vi "initCSMs.vi"(7 "Enable building lvlibp?":bool, 8 "error in (no error)":errorcluster, 11 "TestCase in":refnum<class "testcase-CSMAddonLoopSupport.lvclass">) -> (0 "error out":errorcluster, 3 "TestCase out":refnum<class "testcase-CSMAddonLoopSupport.lvclass">)   [LabVIEW 2017, in "testcase-CSMAddonLoopSupport.lvclass"]
uses:
  testcase-CSMAddonLoopSupport.lvclass
  testcase-CSMAddonLoopSupport.lvclass/testcase-CSMAddonLoopSupport.ctl
  CSM/Normal-CSM.vi
  <vilib>/AppBuilder/AB_API_Simple/Build (path).vi
  CSM/Chain1.vi
  CSM/Chain2.vi
  CSM/Chain3.vi
  <vilib>/addons/_JKI Toolkits/VI Tester/TestCase.llb/TestCase.lvclass
  CSM/CSM-Testcase.lvlib
  src/user.lib/_NEVSTOP/Communicable State Machine(CSM)/Communicable State Machine.lvlib
  <vilib>/AppBuilder/AB_API_Simple/NI_App_Builder_API.lvlib
  C:/Program Files (x86)/National Instruments/LabVIEW 2017/vi.lib/addons/_JKI Toolkits/VI Tester/TestCase.llb/TestCase.lvclass
panel:
  out "CSMs":string[](array[string])
  out "Generated files":path[](array[path])
  out "CSMs Left":string[](array[string])
  out "Waited (ms)":u32
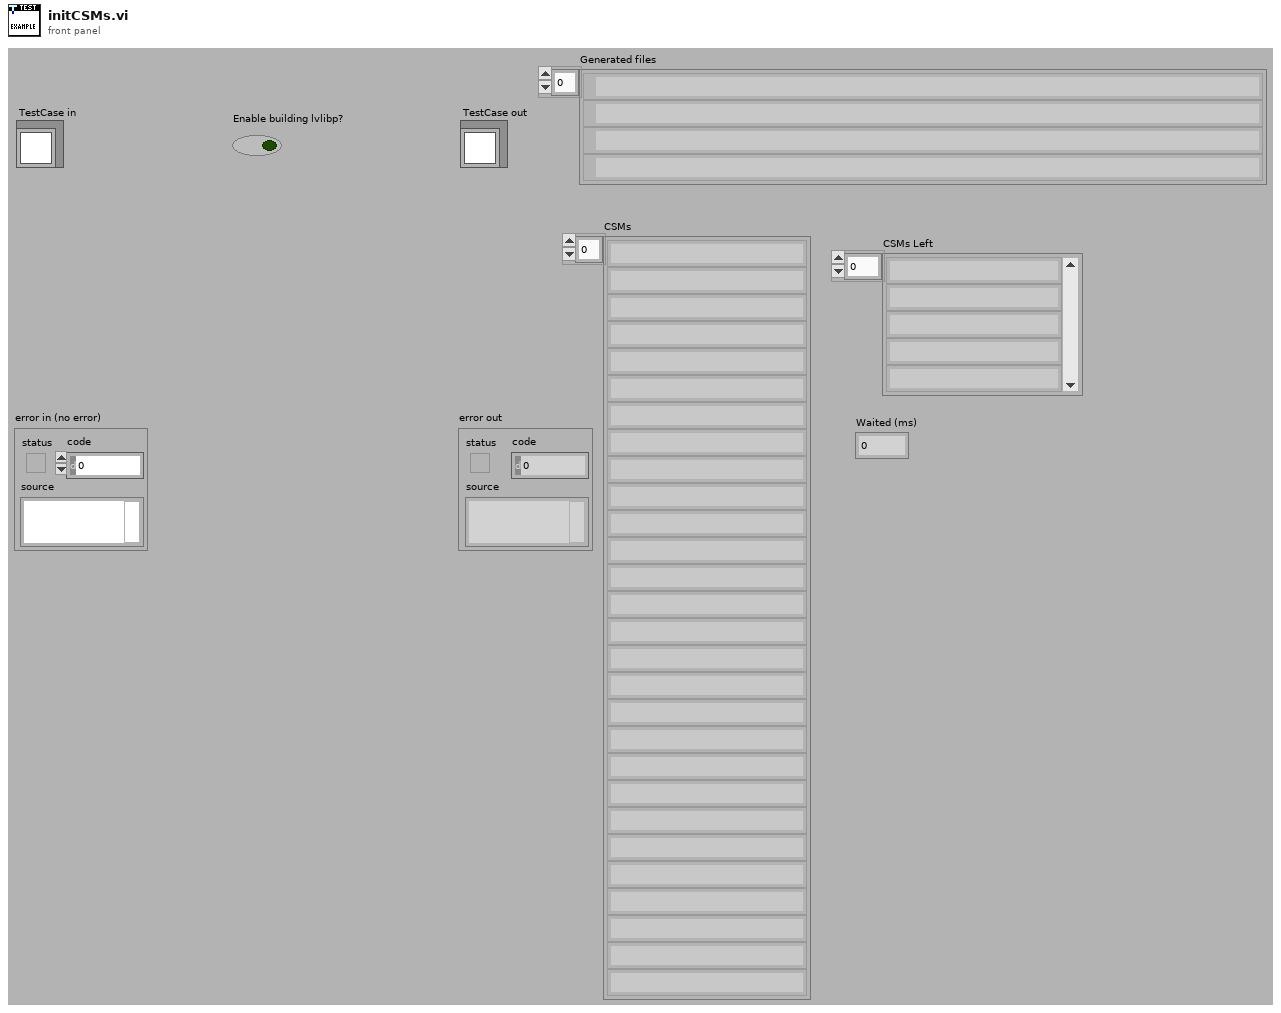
[diagram p1: front panel]
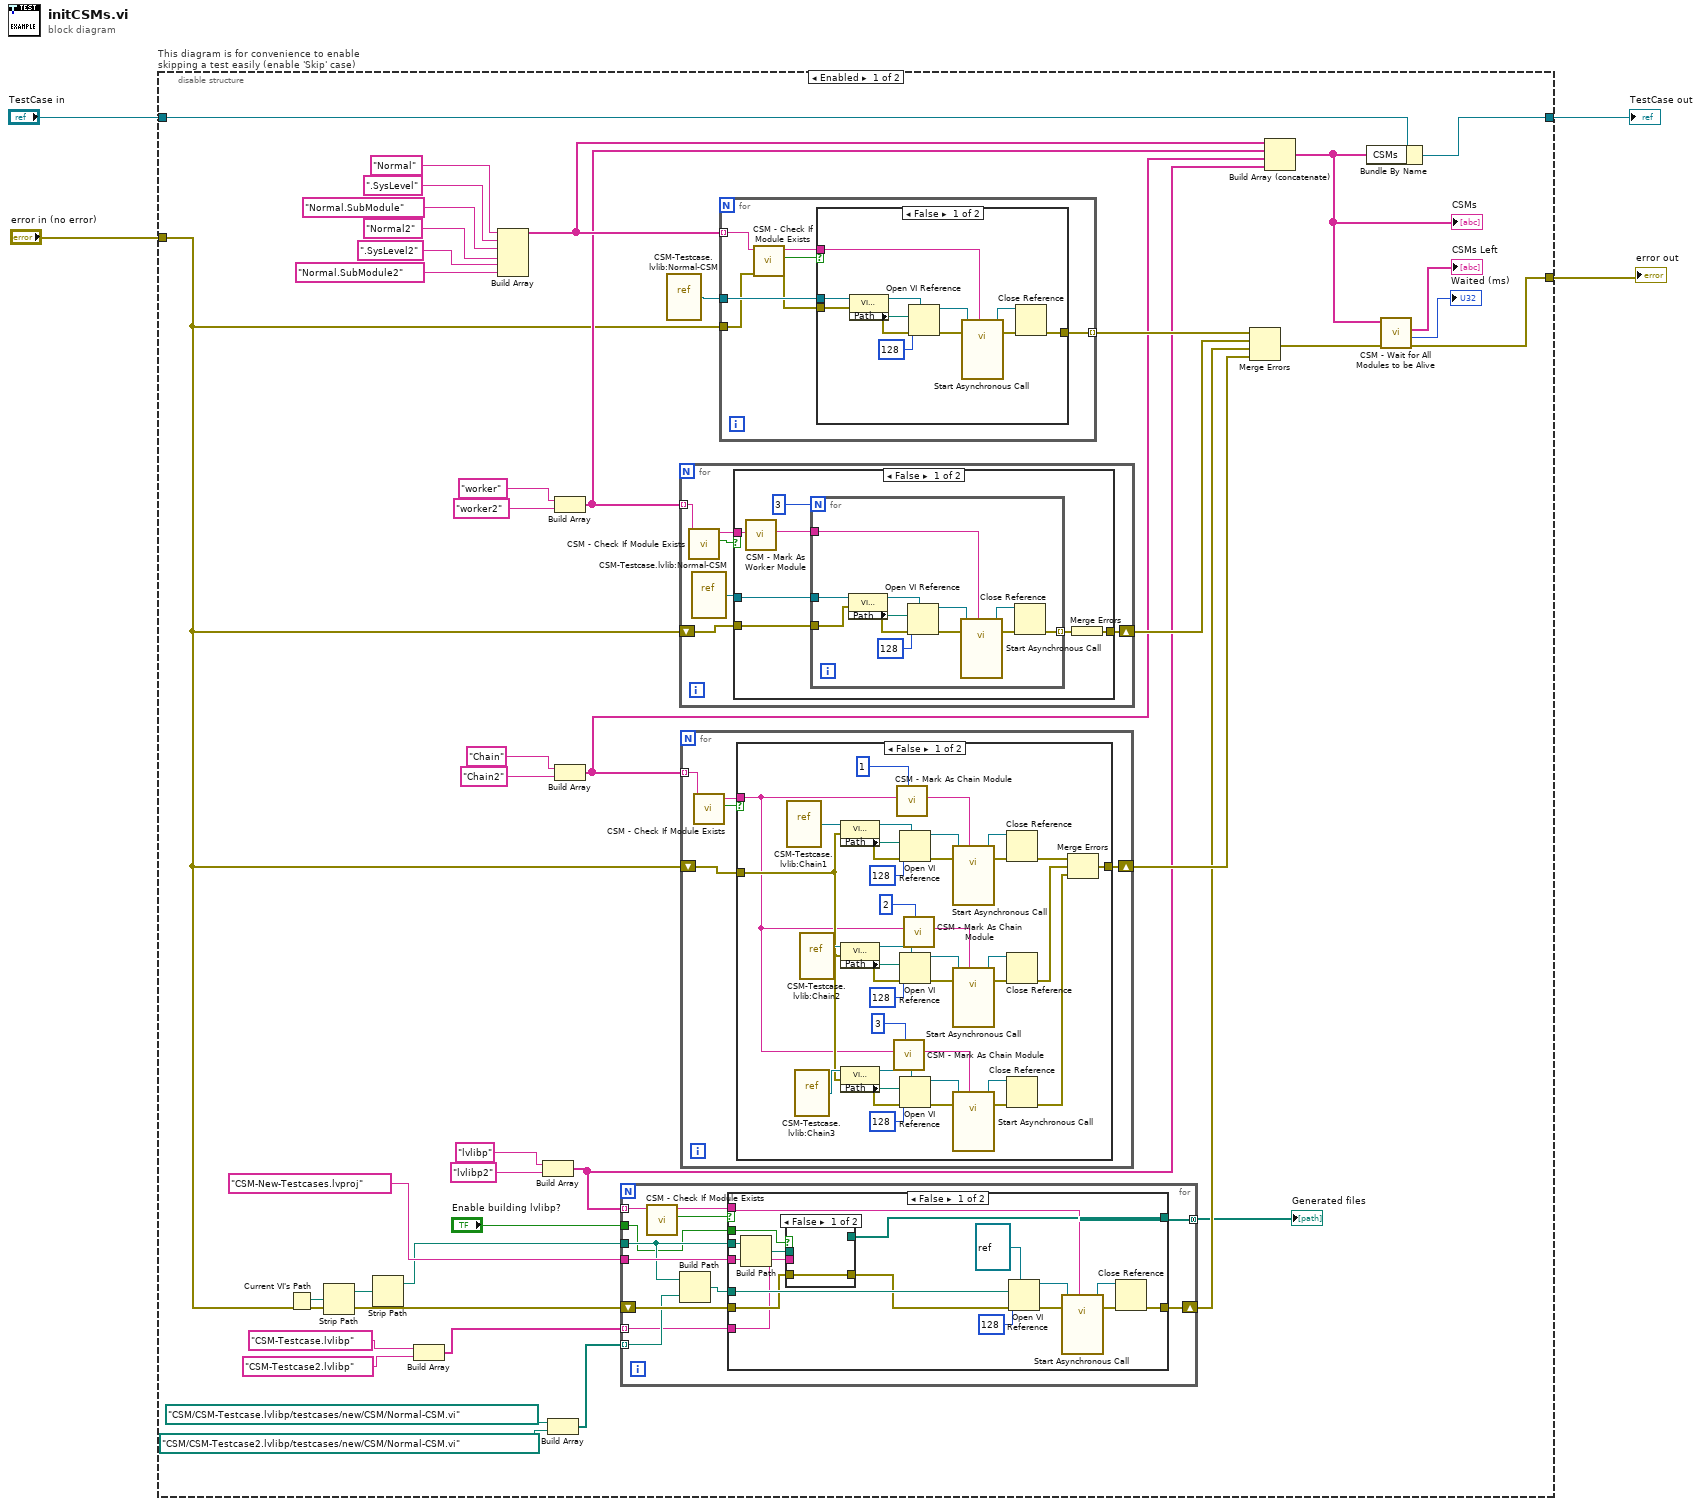
[diagram p0: block diagram]
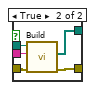
[diagram p2: hidden frame]
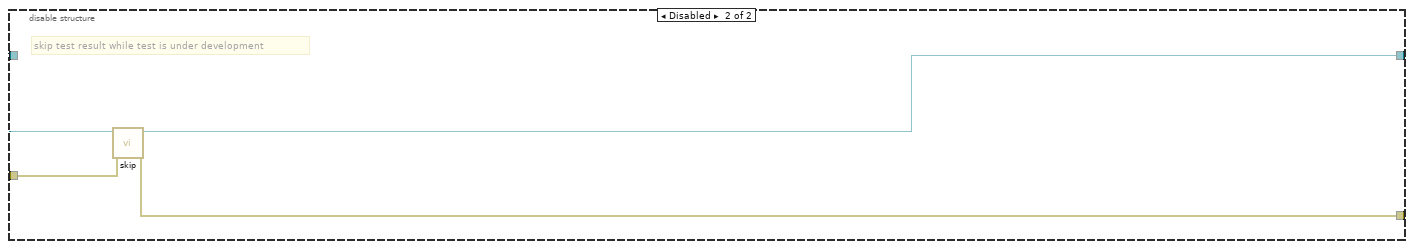
[diagram p7: hidden frame]
diagram:
  n1 = disable-structure "This diagram is for convenience to enable skipping a test easily (enable 'Skip' case)" shown="Enabled" {
    disable-tunnel: "TestCase in" -> [w8 w176]
    disable-tunnel: [w7 w174] -> w2
    disable-tunnel: [w5 w175] -> w1
    disable-tunnel: "error in (no error)" -> [w6 w173]
    frame Enabled {
      n2 = Current VI's Path() -> (path=w41:path)
      n3 = Strip Path(path=w41) -> (stripped path=w42:path)  [unwired: 1 out]
      n4 = Strip Path(path=w42) -> (stripped path=w43:path)  [unwired: 1 out]
      n5 = Build Array("CSM-Testcase.lvlibp" ("Name of build specification (if empty: build all)"), "CSM-Testcase2.lvlibp" ("Name of build specification (if empty: build all)")) -> (w15:string[])
      n6 = Build Array("Normal" ("Name (\"\" to Use UUID)"), ".SysLevel" ("Name (\"\" to Use UUID)"), "Normal.SubModule" ("Name (\"\" to Use UUID)"), "Normal2" ("Name (\"\" to Use UUID)"), ".SysLevel2" ("Name (\"\" to Use UUID)"), "Normal.SubModule2" ("Name (\"\" to Use UUID)")) -> (w37:string[])
      n7 = Build Array("lvlibp" ("Name (\"\" to Use UUID)"), "lvlibp2" ("Name (\"\" to Use UUID)")) -> (w21:string[])
      n8 = Build Array(path "CSM/CSM-Testcase.lvlibp/testcases/new/CSM/Normal-CSM.vi" ("vi path"), path "CSM/CSM-Testcase2.lvlibp/testcases/new/CSM/Normal-CSM.vi" ("vi path")) -> (w18:path[])
      n9 = Build Array("worker" ("Name (\"\" to Use UUID)"), "worker2" ("Name (\"\" to Use UUID)")) -> (w27:string[])
      n10 = Build Array("Chain" ("Name (\"\" to Use UUID)"), "Chain2" ("Name (\"\" to Use UUID)")) -> (w24:string[])
      n11 = for {
        tunnel: "CSM-New-Testcases.lvproj" ("name or relative path") -> [w55]
        tunnel: w43 -> [w50]
        shift-right: [w54] -> w40
        shift-left: w6 -> [w56]
        tunnel: w21 -> [w52] mode=indexing
        tunnel: w18 -> [w51] mode=indexing
        tunnel: w15 -> [w48] mode=indexing
        tunnel: [w47] -> w14 mode=concatenating
        tunnel: "Enable building lvlibp?" -> [w46]
        n12 = call "CSM - Check If Module Exists.vi"("CSM Name"=w52) -> ("Exist?"=w57:bool, "CSM Name (Dup)"=w53:string)  [unwired: 8 in, 1 out]
        n13 = Build Path(base path=w50, name or relative path=w51) -> (appended path=w49:path)
        n14 = case shown="False" w57 {
          tunnel: [w74 w81] -> w54
          tunnel: w49 -> [w67 _]
          tunnel: w50 -> [w66 _]
          tunnel: w55 -> [w64 _]
          tunnel: w53 -> [w63 _]
          tunnel: w56 -> [w62 w81]
          tunnel: w48 -> [w60 _]
          tunnel: [w59 _] -> w47
          tunnel: w46 -> [w58 _]
          frame False {
            n15 = Build Path(base path=w66, name or relative path=w64) -> (appended path=w65:path)
            n16 = case shown="False" w58 {
              tunnel: w65 -> [_ w80]
              tunnel: w62 -> [w75 w79]
              tunnel: [w75 w78] -> w61
              tunnel: w60 -> [_ w77]
              tunnel: [_ w76] -> w59
              frame False {
              }
              frame True {
                n17 = call-poly <vilib>:"Build.vi"("error in (no error)"=w79, "Name of build specification (if empty: build all)"=w77, "Path to project"=w80) -> ("error out"=w78:errorcluster, "Generated files"=w76:path[])  [unwired: 7 in]
              }
            }
            n18 = Open VI Reference(type specifier VI Refnum (for type only)=refnum<vi> refnum ("reference out"), vi path=w67, options=128, error in (no error)=w61) -> (vi reference=w70:refnum<vi>, error out=w72:errorcluster)  [unwired: 2 in]
            n19 = call-by-ref "Start Asynchronous Call"(reference=w70, error in=w72, "Name (\"\" to Use UUID)"=w63) -> (reference out=w69:refnum<vi>, error out=w71:errorcluster)  [unwired: 11 in]
            n20 = Close Reference(reference=w69, error in (no error)=w71) -> (error out=w74:errorcluster)
          }
          frame True {
          }
        }
      }
      "Generated files" <- w14
      n21 = vi-ref "CSM-Testcase.lvlib:Normal-CSM.vi"() -> (w33:refnum<vi>)
      n22 = for {
        shift-right: [w129] -> w39
        shift-left: w6 -> [w132]
        tunnel: w27 -> [w128] mode=indexing
        n23 = call "CSM - Check If Module Exists.vi"("CSM Name"=w128) -> ("Exist?"=w131:bool, "CSM Name (Dup)"=w130:string)  [unwired: 8 in, 1 out]
        n24 = vi-ref "CSM-Testcase.lvlib:Normal-CSM.vi"() -> (w127:refnum<vi>)
        n25 = case shown="False" w131 {
          tunnel: w127 -> [w139 _]
          tunnel: [w133 w152] -> w129
          tunnel: w132 -> [w135 w152]
          tunnel: w130 -> [w134 _]
          frame False {
            n26 = call "CSM - Mark As Worker Module.vi"("CSM Name"=w134) -> ("CSM Name (Marked As Worker)"=w136:string)  [unwired: 9 in]
            n27 = for {
              N: 3 -> [_]
              tunnel: w139 -> [w143]
              tunnel: w136 -> [w142]
              tunnel: [w141] -> w137 mode=indexing
              tunnel: w135 -> [w140]
              n28 = property class="VI (strict)"(reference=w143, error in=w140) -> (reference out=w149:refnum<vi>, error out=w147:errorcluster, "Path"=w146:path)
              n29 = Open VI Reference(type specifier VI Refnum (for type only)=w149, vi path=w146, options=128, error in (no error)=w147) -> (vi reference=w145:refnum<vi>, error out=w150:errorcluster)  [unwired: 2 in]
              n30 = call-by-ref "Start Asynchronous Call"(reference=w145, error in=w150, "Name (\"\" to Use UUID)"=w142) -> (reference out=w144:refnum<vi>, error out=w148:errorcluster)  [unwired: 11 in]
              n31 = Close Reference(reference=w144, error in (no error)=w148) -> (error out=w141:errorcluster)
            }
            n32 = Merge Errors(w137) -> (w133:errorcluster)
          }
          frame True {
          }
        }
      }
      n33 = for {
        shift-right: [w84] -> w45
        shift-left: w6 -> [w86]
        tunnel: w24 -> [w82] mode=indexing
        n34 = call "CSM - Check If Module Exists.vi"("CSM Name"=w82) -> ("Exist?"=w85:bool, "CSM Name (Dup)"=w83:string)  [unwired: 8 in, 1 out]
        n35 = case shown="False" w85 {
          tunnel: [w89 w126] -> w84
          tunnel: w86 -> [w88 w126]
          tunnel: w83 -> [w87 _]
          frame False {
            n36 = vi-ref "CSM-Testcase.lvlib:Chain1.vi"() -> (w125:refnum<vi>)
            n37 = vi-ref "CSM-Testcase.lvlib:Chain3.vi"() -> (w107:refnum<vi>)
            n38 = vi-ref "CSM-Testcase.lvlib:Chain2.vi"() -> (w108:refnum<vi>)
            n39 = property class="VI (strict)"(reference=w125, error in=w88) -> (reference out=w122:refnum<vi>, error out=w120:errorcluster, "Path"=w119:path)
            n40 = property class="VI (strict)"(reference=w108, error in=w88) -> (reference out=w111:refnum<vi>, error out=w113:errorcluster, "Path"=w114:path)
            n41 = property class="VI (strict)"(reference=w107, error in=w88) -> (reference out=w104:refnum<vi>, error out=w102:errorcluster, "Path"=w101:path)
            n42 = call "CSM - Mark As Chain Module.vi"("Order"=3, "CSM Name"=w87) -> ("CSM Name (Marked As Chain)"=w95:string)  [unwired: 8 in]
            n43 = call "CSM - Mark As Chain Module.vi"("Order"=1, "CSM Name"=w87) -> ("CSM Name (Marked As Chain)"=w93:string)  [unwired: 8 in]
            n44 = Open VI Reference(type specifier VI Refnum (for type only)=w122, vi path=w119, options=128, error in (no error)=w120) -> (vi reference=w118:refnum<vi>, error out=w123:errorcluster)  [unwired: 2 in]
            n45 = Open VI Reference(type specifier VI Refnum (for type only)=w111, vi path=w114, options=128, error in (no error)=w113) -> (vi reference=w115:refnum<vi>, error out=w110:errorcluster)  [unwired: 2 in]
            n46 = Open VI Reference(type specifier VI Refnum (for type only)=w104, vi path=w101, options=128, error in (no error)=w102) -> (vi reference=w100:refnum<vi>, error out=w105:errorcluster)  [unwired: 2 in]
            n47 = call "CSM - Mark As Chain Module.vi"("Order"=2, "CSM Name"=w87) -> ("CSM Name (Marked As Chain)"=w94:string)  [unwired: 8 in]
            n48 = call-by-ref "Start Asynchronous Call"(reference=w118, error in=w123, "Name (\"\" to Use UUID)"=w93) -> (reference out=w117:refnum<vi>, error out=w121:errorcluster)  [unwired: 11 in]
            n49 = call-by-ref "Start Asynchronous Call"(reference=w115, error in=w110, "Name (\"\" to Use UUID)"=w94) -> (reference out=w116:refnum<vi>, error out=w112:errorcluster)  [unwired: 11 in]
            n50 = call-by-ref "Start Asynchronous Call"(reference=w100, error in=w105, "Name (\"\" to Use UUID)"=w95) -> (reference out=w99:refnum<vi>, error out=w103:errorcluster)  [unwired: 11 in]
            n51 = Close Reference(reference=w117, error in (no error)=w121) -> (error out=w98:errorcluster)
            n52 = Close Reference(reference=w116, error in (no error)=w112) -> (error out=w97:errorcluster)
            n53 = Close Reference(reference=w99, error in (no error)=w103) -> (error out=w96:errorcluster)
            n54 = Merge Errors(w98, w97, w96) -> (w89:errorcluster)
          }
          frame True {
          }
        }
      }
      n55 = for {
        tunnel: w33 -> [w159]
        tunnel: w37 -> [w155] mode=indexing
        tunnel: [w158] -> w38 mode=indexing
        tunnel: w6 -> [w157]
        n56 = call "CSM - Check If Module Exists.vi"("Error In"=w157, "CSM Name"=w155) -> ("error out"=w156:errorcluster, "Exist?"=w153:bool, "CSM Name (Dup)"=w154:string)  [unwired: 7 in]
        n57 = case shown="False" w153 {
          tunnel: w159 -> [w163 _]
          tunnel: [w162 w172] -> w158
          tunnel: w156 -> [w161 w172]
          tunnel: w154 -> [w160 _]
          frame False {
            n58 = property class="VI (strict)"(reference=w163, error in=w161) -> (reference out=w169:refnum<vi>, error out=w167:errorcluster, "Path"=w166:path)
            n59 = Open VI Reference(type specifier VI Refnum (for type only)=w169, vi path=w166, options=128, error in (no error)=w167) -> (vi reference=w165:refnum<vi>, error out=w170:errorcluster)  [unwired: 2 in]
            n60 = call-by-ref "Start Asynchronous Call"(reference=w165, error in=w170, "Name (\"\" to Use UUID)"=w160) -> (reference out=w164:refnum<vi>, error out=w168:errorcluster)  [unwired: 11 in]
            n61 = Close Reference(reference=w164, error in (no error)=w168) -> (error out=w162:errorcluster)
          }
          frame True {
          }
        }
      }
      n62 = Merge Errors(w38, w39, w40, w45) -> (w13:errorcluster)
      n63 = Build Array (concatenate)(w37, w27, w24, w21) -> (w12:string[])
      "CSMs" <- w12
      n64 = Bundle By Name(cluster=w8, "CSMs"=w12) -> (w7:refnum<class "testcase-CSMAddonLoopSupport.lvclass">)
      n65 = call "CSM - Wait for All Modules to be Alive.vi"("Error In"=w13, "CSM Names"=w12) -> ("error out"=w5:errorcluster, "Waited (ms)"=→"Waited (ms)":u32, "CSMs Left"=→"CSMs Left":string[])  [unwired: 7 in]
    }
    frame Disabled {
      # "skip test result while test is under development"
      n66 = call <vilib>:"skip.vi"("error in (no error)"=w173, "TestCase in"=w176) -> ("error out"=w175:errorcluster, "TestCase out"=w174:refnum<class "testcase-CSMAddonLoopSupport.lvclass">)  [unwired: 8 in]
    }
  }
  "error out" <- w1
  "TestCase out" <- w2
